vi "Log Data to File.vi"(7 "First Log Value":bool, 8 "error in":errorcluster, 9 "WiBCI16T Data out":T1 {"Reg Map"."ADS2" format="%x"; "Reg Map"."ADS1" format="%x"}, 10 "file path":path, 11 "Text refnum":refnum<file>) -> (0 "error out":errorcluster)   [LabVIEW 2019, in "Logger.lvlib"]
doc: "This VI uses the TDMS Write function to write data to a TDMS file.\n_____\nBased on DQMH Project Template 6.1.0.94."
uses:
  Logger.lvlib
  Acquisition/WiBCI16T_Data.ctl
  Acquisition/WiBCI16T_Status.ctl
  Acquisition/Reg_Map.ctl
  <vilib>/Utility/file.llb/Write Delimited Spreadsheet (DBL).vi
  Acquisition/Acquisition.lvlib
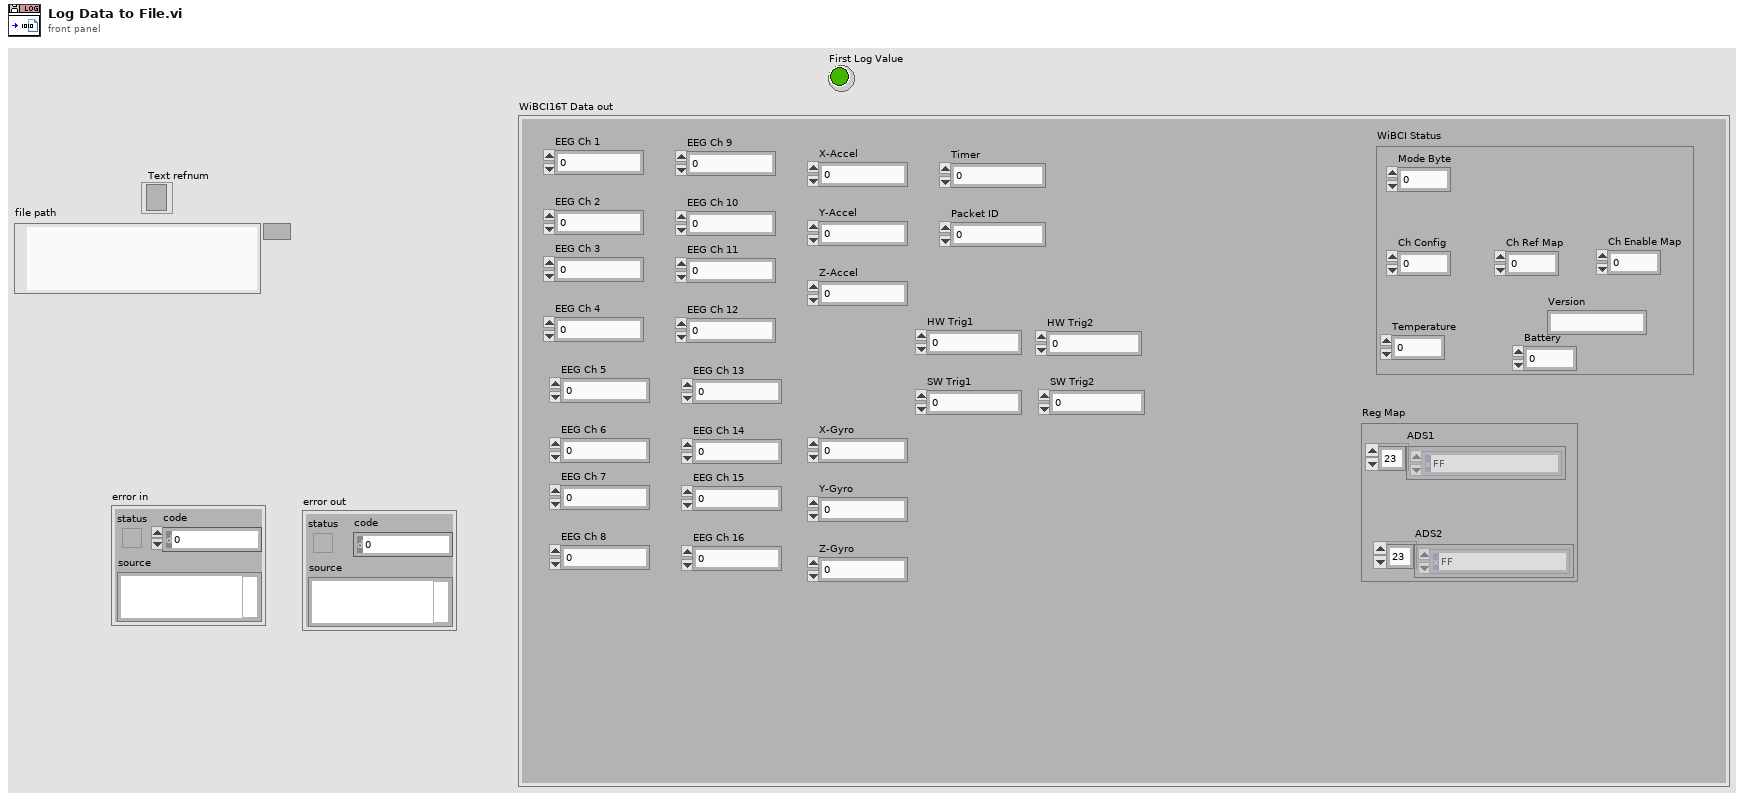
[diagram p1: front panel]
types:
  T1 = typedef "Acquisition.lvlib/WiBCI16T_Data.ctl" = cluster{"EEG Ch 1":dbl, "EEG Ch 2":dbl, "EEG Ch 3":dbl, "EEG Ch 4":dbl, "EEG Ch 5":dbl, "EEG Ch 6":dbl, "EEG Ch 7":dbl, "EEG Ch 8":dbl, "EEG Ch 9":dbl, "EEG Ch 10":dbl, "EEG Ch 11":dbl, "EEG Ch 12":dbl, "EEG Ch 13":dbl, "EEG Ch 14":dbl, "EEG Ch 15":dbl, "EEG Ch 16":dbl, "X-Accel":i16, "Y-Accel":i16, "Z-Accel":i16, "X-Gyro":i16, "Y-Gyro":i16, "Z-Gyro":i16, "Timer":u32, "Packet ID":u32, "HW Trig1":u8, "SW Trig1":i8, "HW Trig2":u8, "SW Trig2":i8, "WiBCI Status":T2, "Reg Map":T3}
  T2 = typedef "Acquisition.lvlib/WiBCI16T_Status.ctl" = cluster{"Mode Byte":u8, "Ch Config":u8, "Ch Ref Map":u16, "Ch Enable Map":u16, "Temperature":sgl, "Battery":u8, "Version":string}
  T3 = typedef "Acquisition.lvlib/Reg_Map.ctl" = cluster{"ADS1":u8[], "ADS2":u8[]}
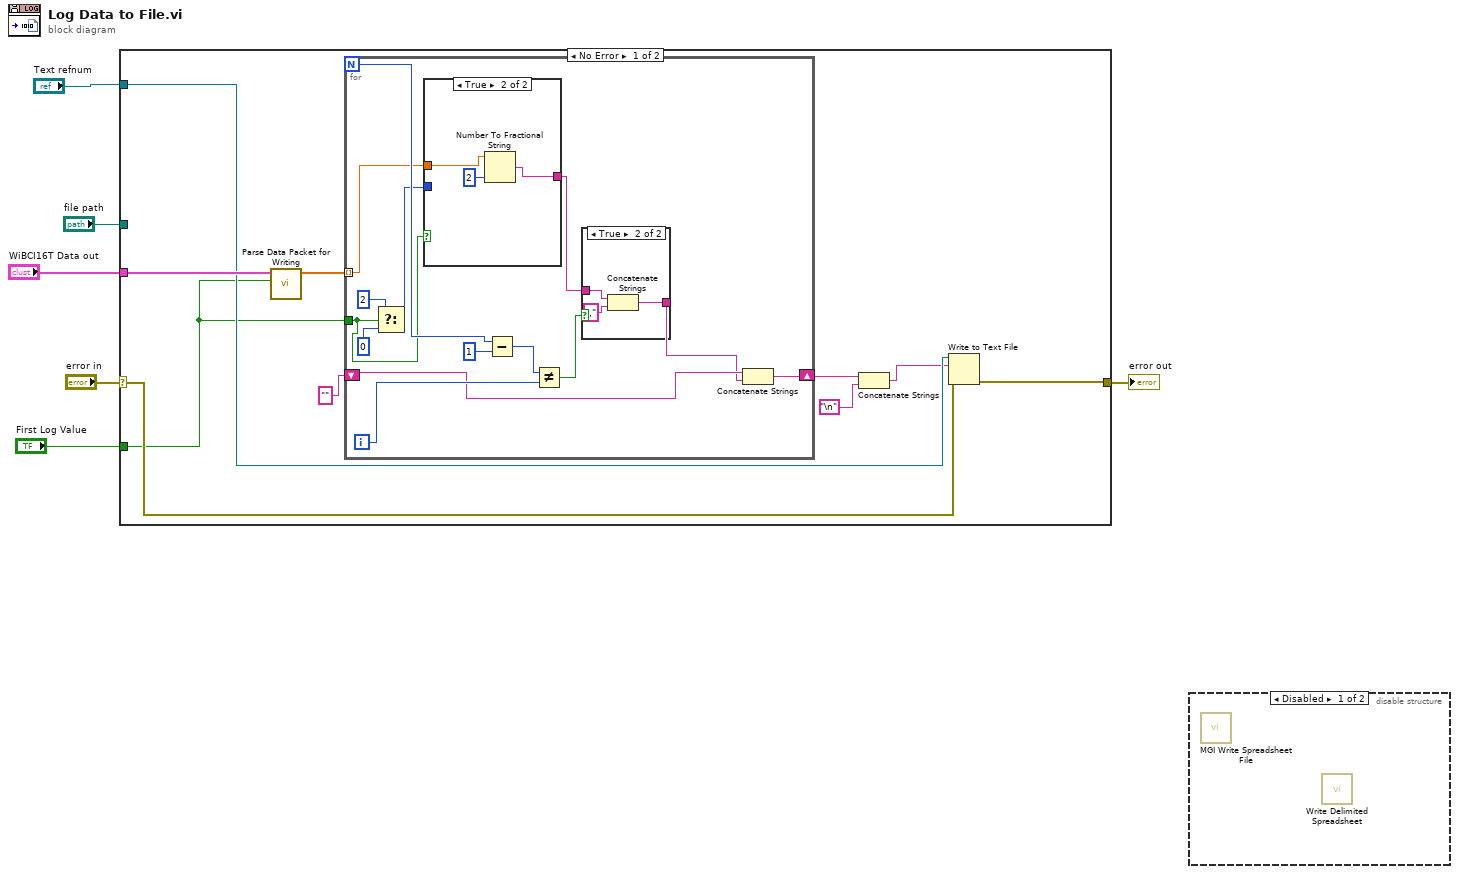
[diagram p0: block diagram]
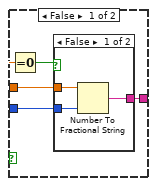
[diagram p3: hidden frame]
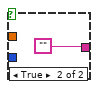
[diagram p4: hidden frame]
diagram:
  n1 = case shown="No Error" "error in" {
    selector: "error in" -> [w13 w46]
    tunnel: [w14 w46] -> w6
    tunnel: "Text refnum" -> [w15 _]
    tunnel: "file path" -> [_ _]
    tunnel: "WiBCI16T Data out" -> [w16 _]
    tunnel: "First Log Value" -> [w10 _]
    frame No Error {
      n2 = call "Parse Data Packet for Writing.vi"("First Log Value in"=w10, "WiBCI16T Data in"=w16) -> ("Array"=w12:dbl[])  [unwired: 9 in]
      n3 = for {
        N -> [w29]
        tunnel: w12 -> [w18] mode=indexing
        shift-right: [w22] -> w9
        shift-left: "" -> [w24]
        tunnel: w10 -> [w17]
        i -> [w26]
        n4 = Select(t=i16 2 ("precision (6)"), s=w17, f=i16 0 ("precision (6)")) -> (s? t:f=w19:i16)
        n5 = case shown="True" w17 {
          tunnel: [w34 w39] -> w30
          tunnel: w19 -> [w33 _]
          tunnel: w18 -> [w32 w41]
          frame False {
            n6 = Equal To 0?(x=w32) -> (x = 0?=w31:bool)
            n7 = case shown="False" w31 {
              tunnel: w32 -> [w37 _]
              tunnel: [w36 ""] -> w34
              tunnel: w33 -> [w35 _]
              frame False {
                n8 = Number To Fractional String(number=w37, precision (6)=w35) -> (F-format string=w36:string)  [unwired: 2 in]
              }
              frame True {
              }
            }
          }
          frame True {
            n9 = Number To Fractional String(number=w41, precision (6)=i16 2) -> (F-format string=w39:string)  [unwired: 2 in]
          }
        }
        n10 = Subtract(x=w29, y=1) -> (x-y=w27:i32)
        n11 = Not Equal?(x=w27, y=w26) -> (x != y?=w25:bool)
        n12 = case shown="True" w25 {
          tunnel: w30 -> [w42 w45]
          tunnel: [w42 w43] -> w23
          frame False {
          }
          frame True {
            n13 = Concatenate Strings(w45, "," ("delimiter (\\t)")) -> (w43:string)
          }
        }
        n14 = Concatenate Strings(w24, w23) -> (w22:string)
      }
      n15 = Concatenate Strings(w9, "\n") -> (w8:string)
      n16 = Write to Text File(file (use dialog)=w15, text=w8, error in=w13) -> (error out=w14:errorcluster)  [unwired: 1 in, 2 out]
    }
    frame Error {
    }
  }
  "error out" <- w6
  n17 = disable-structure shown="Disabled" {
    frame Disabled {
      n18 = call <userlib>:"MGI Write Spreadsheet File.vi"() -> ()  [unwired: 8 in, 4 out]
      n19 = call-poly <vilib>:"Write Delimited Spreadsheet.vi"() -> ()  [unwired: 14 in, 2 out]
    }
    frame Enabled {
    }
  }
